vi "Impedance Equivalent Circuit Converter.vi"(0 "major in":dbl, 1 "u(major) in":dbl, 2 "minor in":dbl, 3 "u(minor) in":dbl, 4 "f [Hz]":dbl, 5 "error in (no error)":errorcluster, 6 "type in":T2=enum."Rs-Xs", 8 "type in by string":string, 10 "type out by string":string, 12 "type out":T2=enum."Rs-Xs") -> (14 "major out":dbl, 15 "u(major) out":dbl, 16 "minor out":dbl, 17 "u(minor) out":dbl, 18 "type out info":T1, 19 "error out":errorcluster)   [LabVIEW 2020]
doc: "Impedance equivalent circuit connection converter. Identify input and output types either by type id or type string."
uses:
  Impedance Equivalent Circuit.ctl
  Impedance Equivalent Circuit Type Info.ctl
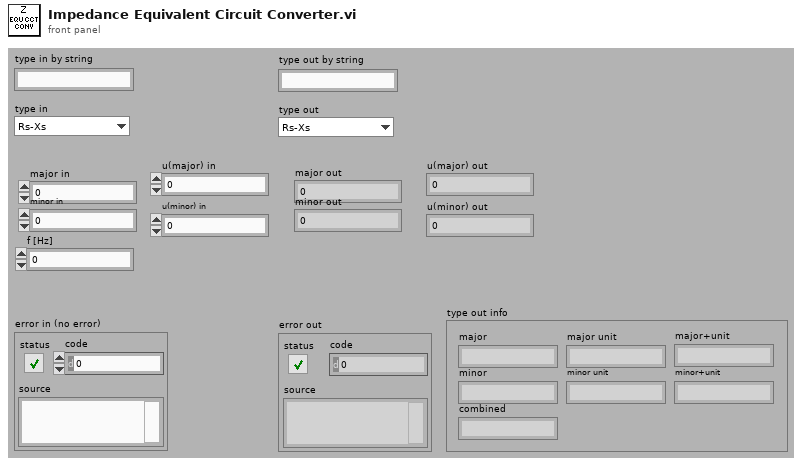
[diagram p1: front panel]
types:
  T1 = typedef "Impedance Equivalent Circuit Type Info.ctl" = cluster{"major":string, "major unit":string, "minor":string, "minor unit":string, "combined":string, "major+unit":string, "minor+unit":string}
  T2 = typedef "Impedance Equivalent Circuit.ctl" = enum16{"Keep original", "Rs-Xs", "Gp-Bp", "Z-phid", "Z-phir", "Y-phid", "Y-phir", "Cp-D", "Cp-Q", "Cp-Rp", "Cp-Gp", "Cs-D", "Cs-Q", "Cs-Rs", "Ls-Rs", "Ls-Q", "Rs-Tau", "Rp-Tau", "Lp-Q", "Lp-Rp"}
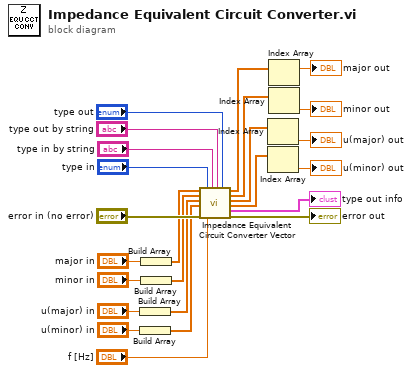
[diagram p0: block diagram]
diagram:
  n1 = Build Array("u(major) in") -> (w10:dbl[])
  n2 = Build Array("u(minor) in") -> (w9:dbl[])
  n3 = Build Array("major in") -> (w12:dbl[])
  n4 = Build Array("minor in") -> (w11:dbl[])
  n5 = call "Impedance Equivalent Circuit Converter Vector.vi"("major in"=w12, "u(major) in"=w11, "minor in"=w10, "u(minor) in"=w9, "error in (no error)"="error in (no error)", "type in"="type in", "f scalar [Hz]"="f [Hz]", "type in by string"="type in by string", "type out by string"="type out by string", "type out"="type out") -> ("major out"=w8:dbl[], "u(major) out"=w6:dbl[], "minor out"=w4:dbl[], "u(minor) out"=w3:dbl[], "type out info"=→"type out info":T1, "error out"=→"error out":errorcluster)  [unwired: 4 in]
  n6 = Index Array(array=w4) -> (element=→"u(major) out":dbl)  [unwired: 1 in]
  n7 = Index Array(array=w3) -> (element=→"u(minor) out":dbl)  [unwired: 1 in]
  n8 = Index Array(array=w8) -> (element=→"major out":dbl)  [unwired: 1 in]
  n9 = Index Array(array=w6) -> (element=→"minor out":dbl)  [unwired: 1 in]
